vi "EncoderPositionCalc.vi"(9 "PositionTarget(in)":dbl, 10 "Wheel Size(in)":dbl=4.0, 11 "EncoderCount/Revolution":dbl=4096.0) -> (3 "PostionTarget(Counts)":i32)   [LabVIEW 2017]
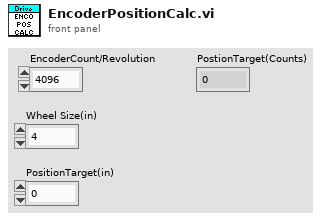
[diagram p1: front panel]
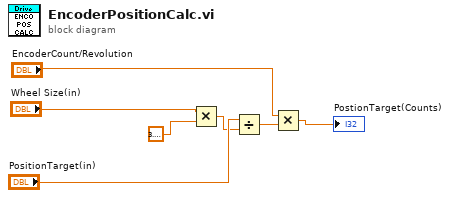
[diagram p0: block diagram]
diagram:
  n1 = Multiply(x="Wheel Size(in)", y=3.141592653589793) -> (x*y=w1:dbl)
  n2 = Divide(x="PositionTarget(in)", y=w1) -> (x/y=w5:dbl)
  n3 = Multiply(x="EncoderCount/Revolution", y=w5) -> (x*y=→"PostionTarget(Counts)":dbl)
